vi "file version adapter.vi"(7 "Type":variant, 8 "Error in":errorcluster caption="Error in (no error)", 11 "Variant":variant) -> (0 "Error out":errorcluster, 3 "Variant (dup)":variant)   [LabVIEW 2017, in "TagDB.lvlib"]
uses:
  TagDB.lvlib
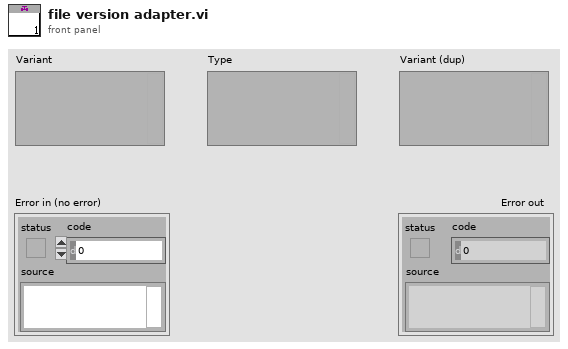
[diagram p1: front panel]
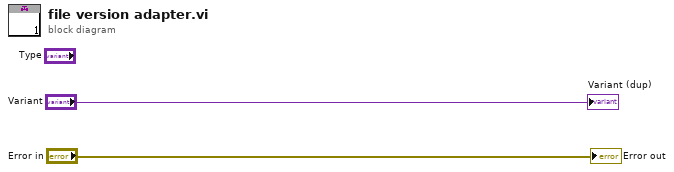
[diagram p0: block diagram]
diagram:
  "Error out" <- "Error in"
  "Variant (dup)" <- "Variant"
